vi "Refresh Waveform.vi"(8 "error in":errorcluster, 10 "Waveform":waveform(dbl)[](array[waveform]), 11 "Report Viewer in":refnum<class "Report Viewer.lvclass">) -> (0 "error out":errorcluster, 3 "Report Viewer out":refnum<class "Report Viewer.lvclass">)   [LabVIEW 2019, in "Report Viewer.lvlib" / "Report Viewer.lvclass"]
uses:
  Library/Report Viewer.lvclass
  Library/Report Viewer.lvclass/Report Viewer.ctl
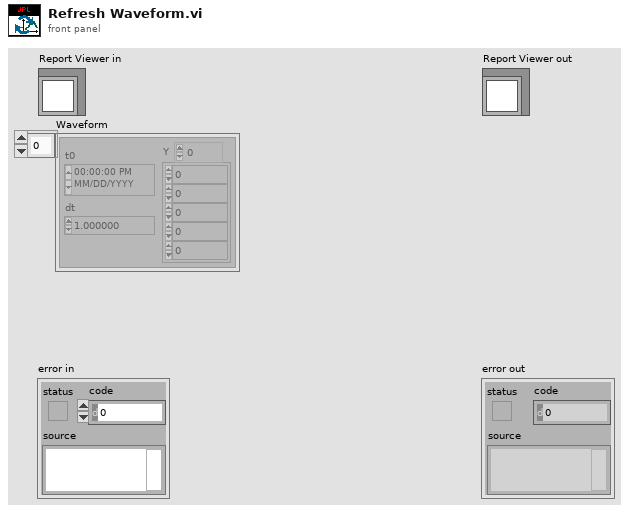
[diagram p1: front panel]
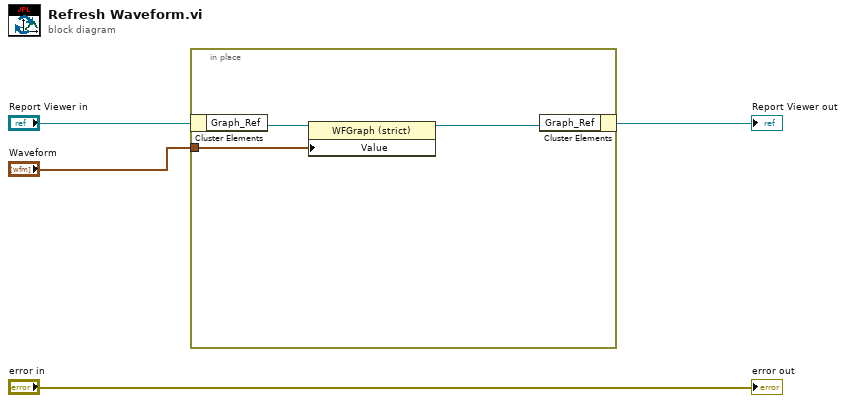
[diagram p0: block diagram]
diagram:
  n1 = in-place {
    in-place-border: "Waveform" -> [w5]
    n2 = in-place-cluster #1("Report Viewer in") -> ("Graph_Ref"=w7:refnum<vi>)
    n3 = property class="WFGraph (strict)"(reference=w7, "Value"=w5) -> (reference out=w6:refnum<vi>)  [unwired: 1 in, 1 out]
    n4 = in-place-cluster #1("Graph_Ref"=w6) -> (→"Report Viewer out":refnum<class "Report Viewer.lvclass">)
  }
  "error out" <- "error in"
